vi "lfield_set_experiment.vi"(8 "error in (no error)":errorcluster, 10 "experiment_name":string, 11 "lightfield_class in":refnum<class "lightfield_class.lvclass">) -> (0 "error out":errorcluster, 3 "lightfield_class out":refnum<class "lightfield_class.lvclass">)   [LabVIEW 2015, in "lightfield_class.lvclass"]
uses:
  lightfield_class.lvclass
  lightfield_class.lvclass/lightfield_class.ctl
  lightfield-automation-labview/LightField Automation.lvclass
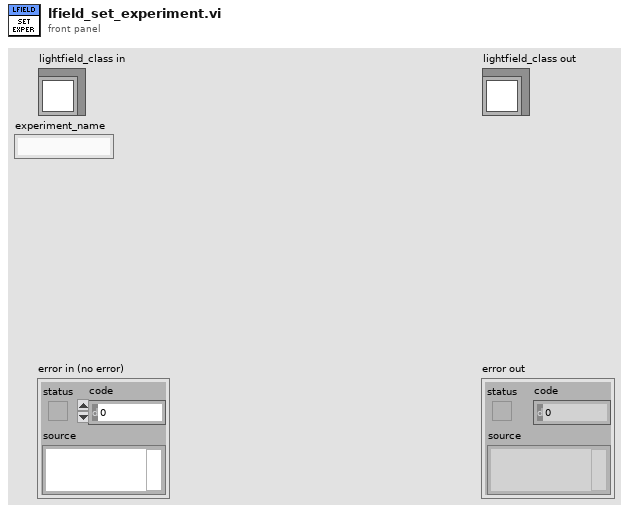
[diagram p1: front panel]
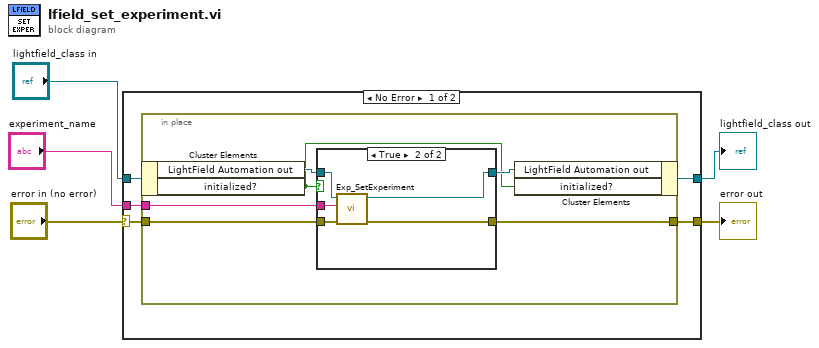
[diagram p0: block diagram]
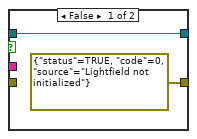
[diagram p2: hidden frame]
diagram:
  n1 = case shown="No Error" "error in (no error)" {
    selector: "error in (no error)" -> [w9 w25]
    tunnel: [w8 w25] -> w4
    tunnel: [w6 w24] -> w2
    tunnel: "lightfield_class in" -> [w7 w24]
    tunnel: "experiment_name" -> [w10 _]
    frame No Error {
      n2 = in-place {
        in-place-border: w10 -> [w14]
        in-place-border: w9 -> [w13]
        in-place-border: [w12] -> w8
        n3 = in-place-cluster #1(w7) -> ("LightField Automation out"=w16:refnum<class "LightField Automation.lvclass">, "initialized?"=w11:bool)
        n4 = case shown="True" w11 {
          tunnel: w16 -> [w17 w23]
          tunnel: [w17 w22] -> w15
          tunnel: w14 -> [_ w21]
          tunnel: w13 -> [_ w20]
          tunnel: [errorcluster {"status"=TRUE, "code"=0, "source"="Lightfield not initialized"} ("error out") w19] -> w12
          frame False {
          }
          frame True {
            n5 = call "Exp_SetExperiment.vi"("error in (no error)"=w20, "ExperimentName"=w21, "LightField Automation in"=w23) -> ("error out"=w19:errorcluster, "LightField Automation out"=w22:refnum<class "LightField Automation.lvclass">)  [unwired: 7 in]
          }
        }
        n6 = in-place-cluster #1("LightField Automation out"=w15, "initialized?"=w11) -> (w6:refnum<class "lightfield_class.lvclass">)
      }
    }
    frame Error {
    }
  }
  "error out" <- w4
  "lightfield_class out" <- w2
